vi "Write States.vi"(8 "error in (no error)":errorcluster, 10 "States":T1, 11 "DefendAreaTactic in":refnum<class "DefendAreaTactic.lvclass">) -> (0 "error out":errorcluster, 3 "DefendAreaTactic out":refnum<class "DefendAreaTactic.lvclass">)   [LabVIEW 2024, in "DefendAreaTactic.lvclass"]
uses:
  DefendAreaTactic.lvclass
  DefendAreaTacticStates.ctl
  DefendAreaTactic.lvclass/DefendAreaTactic.ctl
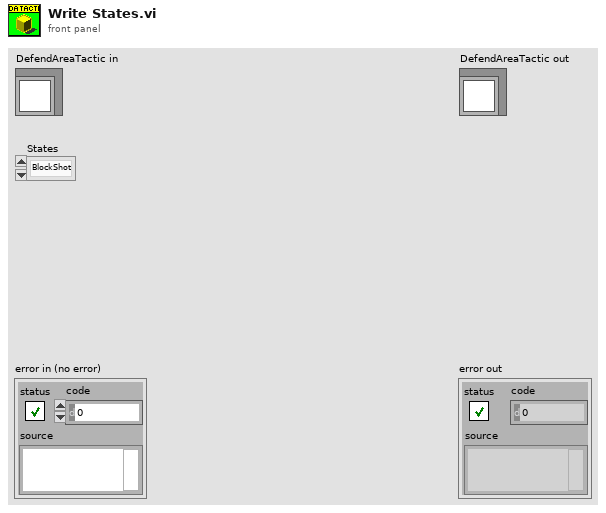
[diagram p1: front panel]
types:
  T1 = typedef "DefendAreaTactic.lvclass/DefendAreaTacticStates.ctl" = enum16{"BlockShot", "BlockPossibleShot", "CoverOneTouchShot", "BallInKeeperArea", "Exit"}
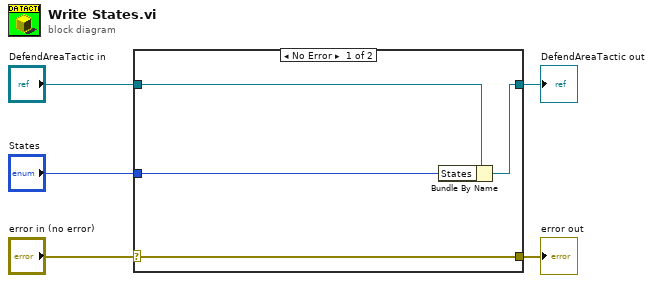
[diagram p0: block diagram]
diagram:
  n1 = case shown="No Error" "error in (no error)" {
    selector: "error in (no error)" -> [w9 w10]
    tunnel: [w9 w10] -> w4
    tunnel: [w7 w11] -> w2
    tunnel: "DefendAreaTactic in" -> [w8 w11]
    tunnel: "States" -> [w6 _]
    frame No Error {
      n2 = Bundle By Name(cluster=w8, "States"=w6) -> (w7:refnum<class "DefendAreaTactic.lvclass">)
    }
    frame Error {
    }
  }
  "error out" <- w4
  "DefendAreaTactic out" <- w2
